vi "Main.vi"() -> ()   [LabVIEW 2018]
doc: "Copyright (c) 2019, Labvolution Limited - www.labvolution.com\n\nThis software is distributed under the BSD 3-Clause License. For the full license please the LICENSE file or visit www.labvolution.com/license"
uses:
  callback-system-exec/callback-system-exec.lvlib
panel:
  out "Exit":bool
  in  "Execute command":bool
  out "Standard Error":string
  out "Standard Out":string
  in  "Working directory":path
  in  "Command":string
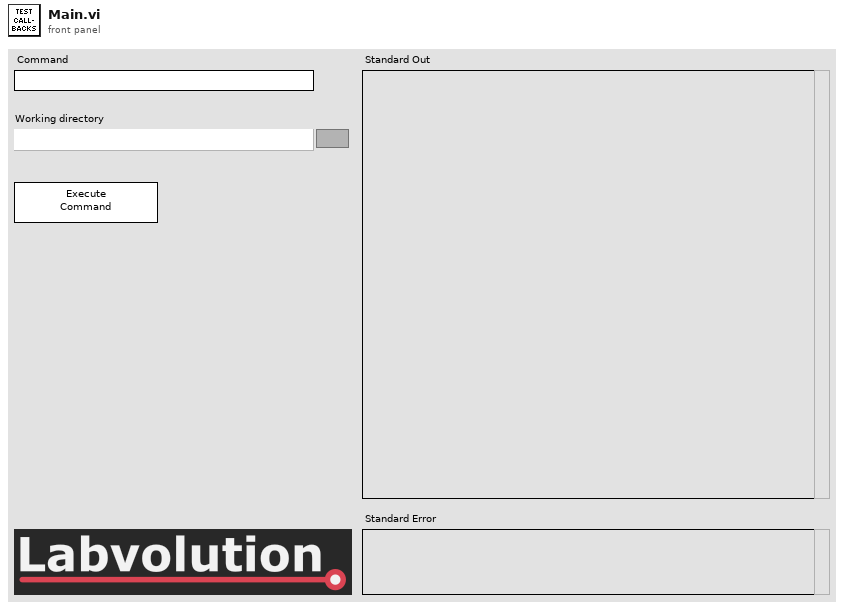
[diagram p1: front panel]
types:
  T1 = cluster{"Standard Out UE":refnum<user-event>, "Standard Error UE":refnum<user-event>, "Exited UE":refnum<user-event>}
  T2 = enum32{"invalid app kind", "Development System", "Run Time System", "Student Edition", "Embedded LabVIEW", "Evaluation", "Custom"}
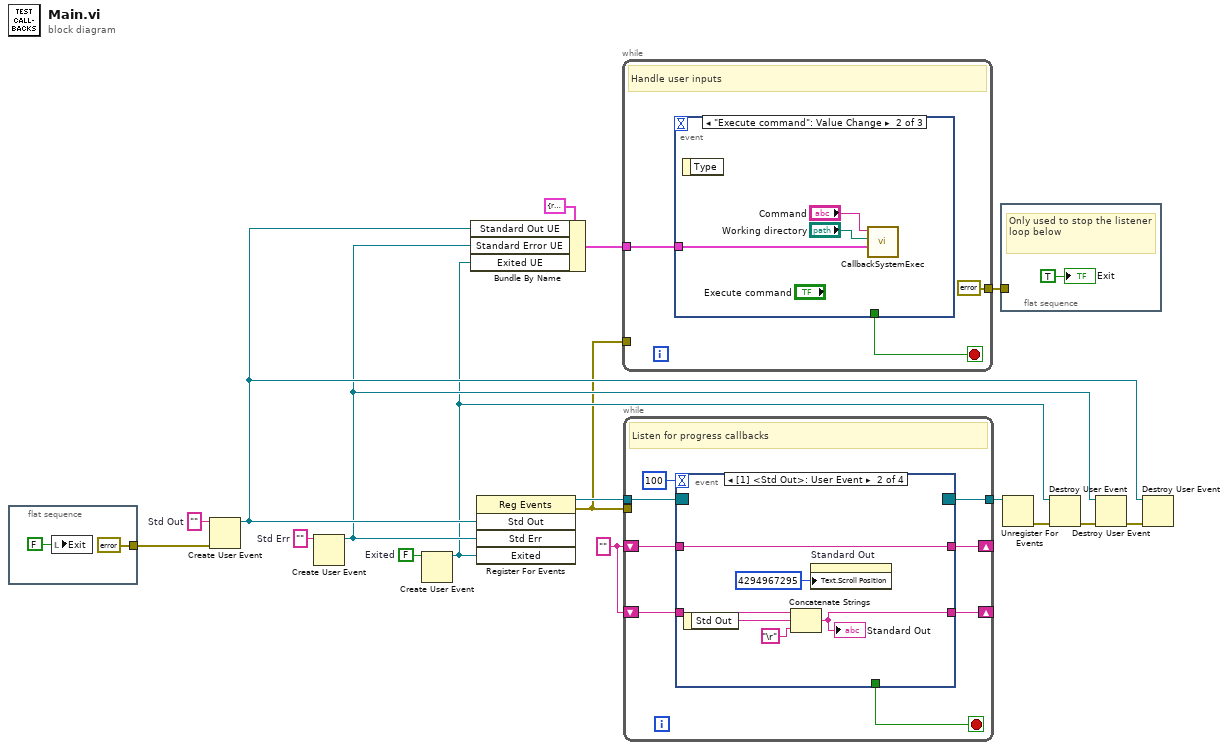
[diagram p0: block diagram]
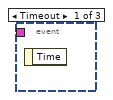
[diagram p2: hidden frame]
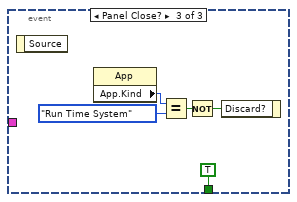
[diagram p3: hidden frame]
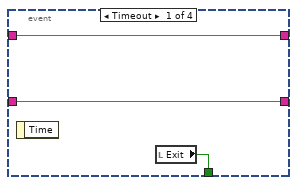
[diagram p4: hidden frame]
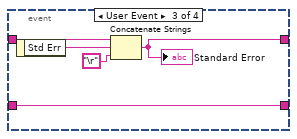
[diagram p5: hidden frame]
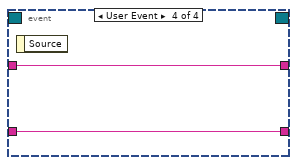
[diagram p6: hidden frame]
diagram:
  w13 = ""
  w17 = FALSE  # Exited
  w16 = ""  # Std Err
  w15 = ""  # Std Out
  n1 = flat-sequence {
    tunnel: [errorcluster {"status"=FALSE, "code"=0, "source"=""} ("error in (no error)")] -> w4
    frame #0 {
      n2 = local write "Exit"(FALSE ("Exit")) -> ()
    }
  }
  n3 = Create User Event(user event datatype=w15, error in=w4) -> (user event=w8:refnum<user-event>)  [unwired: 1 out]
  n4 = Create User Event(user event datatype=w16) -> (user event=w7:refnum<user-event>)  [unwired: 1 in, 1 out]
  n5 = Create User Event(user event datatype=w17) -> (user event=w6:refnum<user-event>)  [unwired: 1 in, 1 out]
  n6 = Bundle By Name(cluster=T1 {"Standard Out UE"=refnum, "Standard Error UE"=refnum, "Exited UE"=refnum} ("Caller Events"), "Standard Out UE"=w8, "Standard Error UE"=w7, "Exited UE"=w6) -> (w1:T1)
  n7 = register-events(w8, w7, w6) -> (reference out=w5:refnum<event-registration>, error out=w3:errorcluster)  [unwired: 2 in]
  n8 = while {
    tunnel: w1 -> [w21]
    tunnel: w3 -> [_]
    tunnel: [errorcluster {"status"=FALSE, "code"=0, "source"=""} ("error in (no error)")] -> w2
    stop <- w22 stop-if-true
    # "Handle user inputs"
    n9 = event shown="[1] \"Execute command\": Value Change" {
      selector: _ -> [_ _ _]
      dyn-events: _ -> [_ _ _]
      timeout: _ -> [_ _ _]
      tunnel: [_ _ TRUE] -> w22
      tunnel: w21 -> [_ w25 _]
      event Timeout {
        n10 = event-data() -> ()  [unwired: 1 in, 1 out]
      }
      event "Execute command": Value Change {
        n11 = event-data() -> ()  [unwired: 1 in, 1 out]
        n12 = call "CallbackSystemExec.vi"("Caller Events"=w25, "Working directory"="Working directory", "Command"="Command") -> ()  [unwired: 6 in, 3 out]
      }
      event Panel Close? {
        n13 = event-data() -> ()  [unwired: 1 in, 1 out]
        n14 = property class="App"() -> ("App.Kind"=w29:T2)  [unwired: 2 in, 2 out]
        n15 = Equal?(x=w29, y=T2."Run Time System") -> (x = y?=w27:bool)
        n16 = Not(x=w27) -> (.not. x?=w26:bool)
        n17 = event-data("Discard?"=w26) -> ()  [unwired: 1 in, 1 out]
      }
    }
  }
  n18 = while {
    tunnel: [w37] -> w9
    shift-right: [w35] -> _
    shift-left: w13 -> [w36]
    shift-right: [w34] -> _
    shift-left: w13 -> [w33]
    tunnel: w5 -> [w32]
    tunnel: w3 -> [_]
    stop <- w38 stop-if-true
    # "Listen for progress callbacks"
    n19 = event shown="[1] <Std Out>: User Event" {
      selector: w32 -> [_ _ _ _]
      dyn-events: [_ _ _ _] -> w37
      timeout: 100 -> [_ _ _ _]
      tunnel: [w39 _ _ _] -> w38
      tunnel: w36 -> [w40 w46 w52 w54]
      tunnel: [w40 w43 w52 w54] -> w35
      tunnel: [w41 w44 w48 w53] -> w34
      tunnel: w33 -> [w41 w44 w50 w53]
      event Timeout {
        n20 = event-data() -> ()  [unwired: 1 in, 1 out]
        n21 = local read "Exit"() -> (w39:bool)
      }
      event User Event {
        n22 = event-data() -> ("Std Out"=w45:string)  [unwired: 1 in]
        n23 = Concatenate Strings(w46, w45, "\r") -> (w43:string)
        "Standard Out" <- w43
        n24 = property on="Standard Out" class="Str"("Text.Scroll Position"=u32 4294967295) -> ()  [unwired: 2 in, 2 out]
      }
      event User Event {
        n25 = event-data() -> ("Std Err"=w49:string)  [unwired: 1 in]
        n26 = Concatenate Strings(w50, w49, "\r") -> (w48:string)
        "Standard Error" <- w48
      }
      event User Event {
        n27 = event-data() -> ()  [unwired: 1 in, 1 out]
      }
    }
  }
  n28 = flat-sequence {
    tunnel: w2 -> [_]
    frame #0 {
      # "Only used to stop the listener loop below"
      "Exit" <- TRUE ("Exit")
    }
  }
  n29 = Unregister For Events(event registration refnum=w9) -> (error out=w10:errorcluster)  [unwired: 1 in]
  n30 = Destroy User Event(user event=w6, error in=w10) -> (error out=w11:errorcluster)
  n31 = Destroy User Event(user event=w7, error in=w11) -> (error out=w12:errorcluster)
  n32 = Destroy User Event(user event=w8, error in=w12) -> ()  [unwired: 1 out]
